vi "Load.vi"(11 "notifier out":refnum<notifier>) -> ()   [LabVIEW 2013, in "main.lvlib"]
uses:
  main.lvlib
panel:
  out "String":string
  out "Horizontal Progress Bar":dbl(slide) scale=0.0..1.0
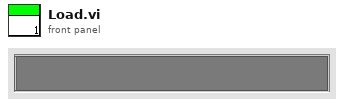
[diagram p1: front panel]
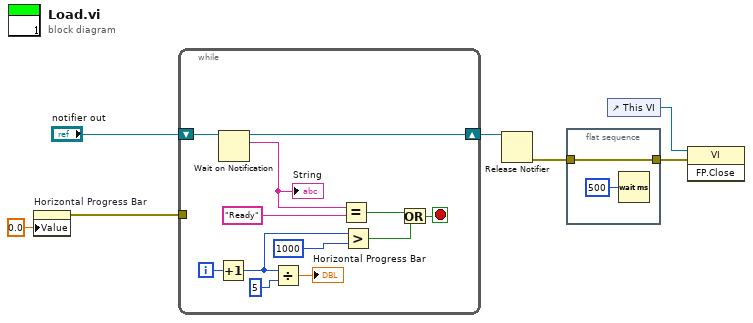
[diagram p0: block diagram]
diagram:
  n1 = property on="Horizontal Progress Bar" class="Slide (strict)"("Value"=0.0 ("Horizontal Progress Bar")) -> (error out=w1:errorcluster)  [unwired: 2 in, 1 out]
  n2 = while {
    shift-right: [w13] -> w7
    shift-left: "notifier out" -> [w14]
    tunnel: w1 -> [_]
    i -> [w15]
    stop <- w8 stop-if-true
    n3 = Increment(x=w15) -> (x+1=w12:i32)
    n4 = Wait on Notification(notifier=w14) -> (notifier out=w13:refnum<notifier>, notification=w17:string)  [unwired: 3 in, 2 out]
    "String" <- w17
    n5 = Divide(x=w12, y=5) -> (x/y=→"Horizontal Progress Bar":dbl)
    n6 = Equal?(x=w17, y="Ready") -> (x = y?=w9:bool)
    n7 = Greater?(x=w12, y=1000) -> (0:w10:bool)
    n8 = Or(x=w9, y=w10) -> (x .or. y?=w8:bool)
  }
  n9 = Release Notifier(notifier=w7) -> (error out=w4:errorcluster)  [unwired: 2 in, 2 out]
  n10 = flat-sequence {
    tunnel: [w20] -> w3
    tunnel: w4 -> [w20]
    frame #0 {
      n11 = Wait (ms)(milliseconds to wait=u32 500) -> ()  [unwired: 1 out]
    }
  }
  n12 = control-ref of="This VI"() -> (w6:refnum<vi>)
  n13 = invoke class="VI" method="FP.Close"(reference=w6, error in=w3) -> ()  [unwired: 1 in, 3 out]
